vi "Get APU List.vi"(8 "error in (no error)":errorcluster, 9 "rio names":string[](array[string]), 11 "Item Ref in":T1 format="%.0x") -> (0 "error out":errorcluster, 2 "ips available":string[](array[string]), 3 "Item Ref out":T1 format="%.0x")   [LabVIEW 2020, in "Engine Simulation Toolkit System Explorer.lvlib"]
uses:
  Engine Simulation Toolkit System Explorer.lvlib
  <vilib>/NI VeriStand/Custom Device API/Custom Device Item Ref.ctl
  Shared/Properties.vi
  <vilib>/NI VeriStand/Custom Device API/Get Item Property (String Array).vi
  <userlib>/_OpenG.lib/array/array.llb/Remove Duplicates from 1D Array (String)__ogtk.vi
  <vilib>/NI VeriStand/Custom Device API/Custom Device API.lvlib
  Shared/Engine Simulation Toolkit Shared.lvlib
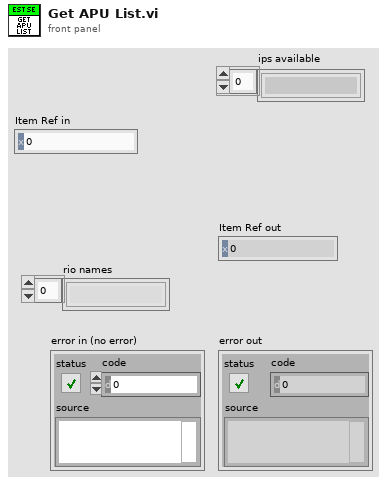
[diagram p1: front panel]
types:
  T1 = typedef "Custom Device API.lvlib/Custom Device Item Ref.ctl" = u64
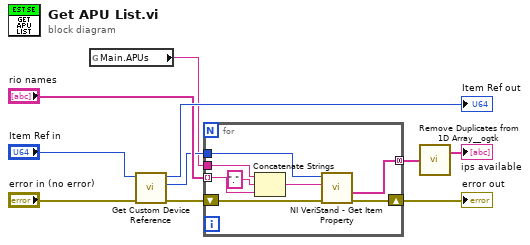
[diagram p0: block diagram]
diagram:
  n1 = global read "Properties.vi" "Main.APUs"() -> (w1:string)
  n2 = call "Get Custom Device Reference.vi"("error in (no error)"="error in (no error)", "Item Ref in"="Item Ref in") -> ("error out"=w5:errorcluster, "Custom Device Ref"=w6:T1, "Item Ref out"=→"Item Ref out":T1)  [unwired: 7 in]
  n3 = for {
    tunnel: "rio names" -> [w14] mode=indexing
    tunnel: w6 -> [w18]
    shift-right: [w16] -> w4
    shift-left: w5 -> [w17]
    tunnel: [w15] -> w3 mode=concatenating
    tunnel: w1 -> [w13]
    n4 = Concatenate Strings(w13, "." ("string"), w14) -> (w11:string)
    n5 = call-poly <vilib>:"NI VeriStand - Get Item Property.vi"("error in (no error)"=w17, "Property Name"=w11, "Item Ref in"=w18) -> ("error out"=w16:errorcluster, "Value"=w15:string[])  [unwired: 5 in, 2 out]
  }
  "error out" <- w4
  n6 = call-poly <userlib>:"Remove Duplicates from 1D Array__ogtk.vi"("Input Array"=w3) -> ("Output Array"=→"ips available":string[])  [unwired: 1 out]
